vi "Load Trigger Model SimpleLoop Template.vi"(0 "VISA resource name":refnum<visa-resource-name>, 1 "Reading Block":u16(ring) items=["Active", "Measure", "Digitize"], 5 "Count":i16, 7 "Delay":dbl, 9 "Reading Buffer":string="defbuffer1", 11 "error in (no error)":errorcluster) -> (4 "VISA resource name out":refnum<visa-resource-name>, 15 "error Out (no error)":errorcluster)   [LabVIEW 2016, in "Keithley DMM7510.lvlib"]
doc: "This VI loads a predefined trigger model configuration that makes continuous measurements for a specified numbers of time."
uses:
  Keithley DMM7510.lvlib
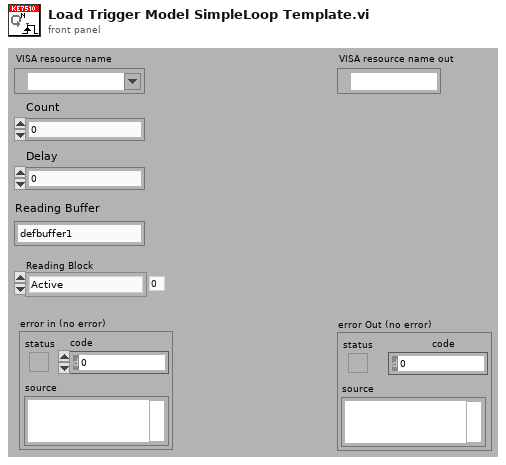
[diagram p1: front panel]
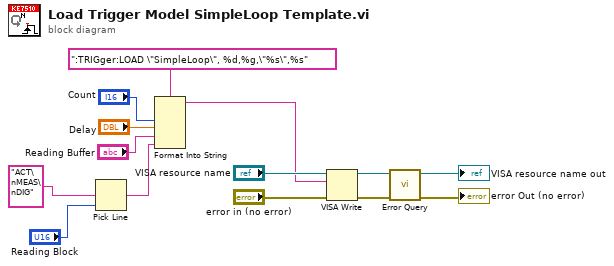
[diagram p0: block diagram]
diagram:
  n1 = Pick Line(multi-line string="ACT\nMEAS\nDIG", line index="Reading Block") -> (output string=w3:string)  [unwired: 1 in]
  n2 = Format Into String(format string=":TRIGger:LOAD \"SimpleLoop\", %d,%g,\"%s\",%s", "Count", "Delay", "Reading Buffer", w3) -> (resulting string=w4:string)  [unwired: 2 in, 1 out]
  n3 = VISA Write(VISA resource name="VISA resource name", write buffer=w4, error in (no error)="error in (no error)") -> (VISA resource name out=w9:refnum<visa-resource-name>, error out=w5:errorcluster)  [unwired: 1 out]
  n4 = call "Error Query.vi"("error in (no error)"=w5, "VISA resource name"=w9) -> ("error out"=→"error Out (no error)":errorcluster, "VISA resource name out"=→"VISA resource name out":refnum<visa-resource-name>)  [unwired: 6 in, 2 out]
